vi "Network Stream Image Host.vi"() -> ()   [LabVIEW 2013]
uses:
  <vilib>/dex/Stream Element Allocation Mode.ctl
  <vilib>/ErrorRing/Error Ring.xnode
panel:
  out "reader url":string
  in  "AVI File Path":path=path "C:/Users/achiu/Desktop/image.png"
  in  "Stop":bool
  in  "Target IP Address":string="localhost"
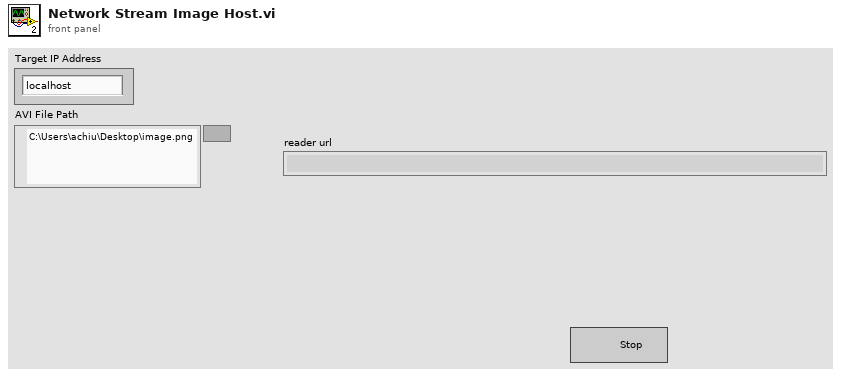
[diagram p1: front panel]
types:
  T1 = typedef "Stream Element Allocation Mode.ctl" = u32
  T2 = typedef "Image Type" = u32
  T3 = typedef "IMAQ Image.ctl" = refnum<image>
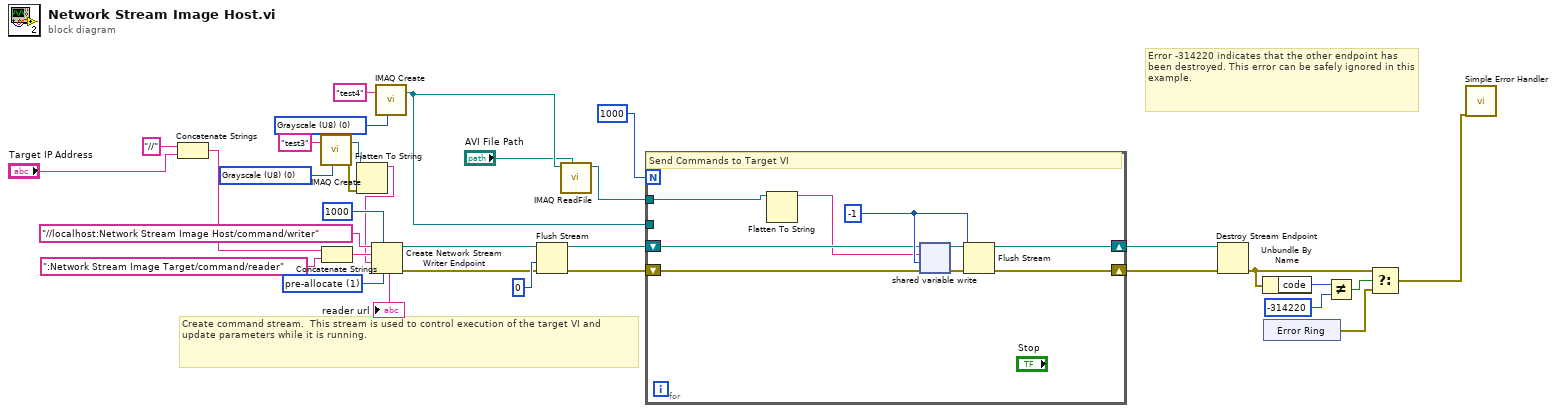
[diagram p0: block diagram]
diagram:
  w4 = T1 1 items=["allocate as needed", "pre-allocate"] ("element allocation mode")
  w9 = T2 0 items=["Grayscale (U8)", "Grayscale (I16)", "Grayscale (SGL)", "Complex (CSG)", "RGB (U32)", "HSL (U32)", "RGB (U64)", "Grayscale (U16)"] ("Image Type")
  w13 = T2 0 items=["Grayscale (U8)", "Grayscale (I16)", "Grayscale (SGL)", "Complex (CSG)", "RGB (U32)", "HSL (U32)", "RGB (U64)", "Grayscale (U16)"] ("Image Type")
  # "Error -314220 indicates that the other endpoint has been destroyed. This error can be safely ignored in this example."
  # "Create command stream.  This stream is used to control execution of the target VI and update parameters while it is running."
  n1 = Concatenate Strings("//" ("reader url"), "Target IP Address") -> (w29:string)
  n2 = call "IMAQ Create"("Image Name"="test3", "Image Type"=w13) -> ("New Image"=w2:T3, "error out"=w3:errorcluster)  [unwired: 3 in]
  n3 = Concatenate Strings(w29, ":Network Stream Image Target/command/reader" ("reader url")) -> (w30:string)
  "reader url" <- w30
  n4 = Flatten To String(anything=w2, error in (no error)=w3) -> (data string=w1:string)  [unwired: 2 in, 2 out]
  n5 = Create Network Stream Writer Endpoint(6:w4, 7:1000 ("writer buffer size"), 9:w1, 10:w30, 11:"//localhost:Network Stream Image Host/command/writer" ("writer name")) -> (0:w11:errorcluster, 3:w12:refnum<k21>)  [unwired: 2 in]
  n6 = call "IMAQ Create"("Image Name"="test4", "Image Type"=w9) -> ("New Image"=w8:T3)  [unwired: 3 in, 1 out]
  n7 = Flush Stream(8:w11, 9:0 ("timeout in ms (-1)"), 11:w12) -> (0:w25:errorcluster, 3:w26:refnum<k21>)  [unwired: 1 in, 1 out]
  n8 = call "IMAQ ReadFile"("File Path"="AVI File Path", "Image"=w8) -> ("Image Out"=w5:T3)  [unwired: 5 in, 4 out]
  n9 = for "Host->Target Command Writer" {
    N: 1000 -> [_]
    shift-right: [w40] -> w22
    shift-left: w25 -> [w36]
    shift-right: [w41] -> w23
    shift-left: w26 -> [w35]
    tunnel: w8 -> [_]
    tunnel: w5 -> [w34]
    w37 = -1 ("timeout in ms (-1)")
    # "Send Commands to Target VI"
    n10 = Flatten To String(anything=w34) -> (data string=w33:string)  [unwired: 3 in, 2 out]
    n11 = shared-variable-write(w35, w36, w33, w37) -> (w39:refnum<k21>, w38:errorcluster)  [unwired: 1 out]
    n12 = Flush Stream(8:w38, 9:w37, 11:w39) -> (0:w40:errorcluster, 3:w41:refnum<k21>)  [unwired: 1 in, 1 out]
  }
  n13 = Destroy Stream Endpoint(8:w22, 11:w23) -> (0:w17:errorcluster)
  n14 = Unbundle By Name(w17) -> ("code"=w18:i32)
  n15 = xnode "Error Ring"() -> ("error out"=w21:errorcluster)
  n16 = Not Equal?(x=w18, y=-314220) -> (x != y?=w20:bool)
  n17 = Select(t=w17, s=w20, f=w21) -> (s? t:f=w15:errorcluster)
  n18 = call <vilib>:"Simple Error Handler.vi"("error in (no error)"=w15) -> ()  [unwired: 4 in, 5 out]
